vi "Producer main.vi"() -> ()   [LabVIEW 2017]
uses:
  Queue define.ctl
  <vilib>/FPGAPlugInAG/cRIO-9065/niLvFpga_Open_cRIO-9065.vi
  <vilib>/rvi/interface/common/dynamic/niFpgaDynamicAddResources.vi
  <vilib>/Utility/error.llb/Error Cluster From Error Code.vi
  <vilib>/rvi/errors/niLvFpgaAdjustHostInterfaceError.vi
  <vilib>/FPGAPlugInAG/Dynamic/niLvFpga_Run_Dynamic.vi
  <vilib>/FPGAPlugInAG/Dynamic/niLvFpga_Abort_Dynamic.vi
  <vilib>/rvi/interface/nirviOpenFPGA/nirviOpenFPGA.xnode
  FPGA Bitfiles/fpgaproject_FPGATarget_fpgamain2_8UW6JkLDP9I.lvbitx
  Fpga.vi
  <vilib>/rvi/interface/nirviMethod/nirviMethod.xnode
  <vilib>/rvi/interface/nirviReadWriteControl/nirviReadWriteControl.xnode
  NiFpgaLv.dll
  <vilib>/rvi/interface/Simulation/niFpgaSimulationCallBeginRW.vi
  <vilib>/FPGAPlugInAG/Dynamic/niLvFpga_StartFifo_Dynamic.vi
  <vilib>/rvi/errors/niLvFpgaMergeErrorWithErrorCode.vi
panel:
  in  "Die Casting?":bool
  out "Voltage Position":cluster{"Speed":dbl[], "Position":dbl[]}(graph)
  out "NO OFFSET Graph":cluster{"Speed":dbl[], "Position":dbl[]}(graph)
  out "OFFSET Graph":cluster{"Speed":dbl[], "Position":dbl[]}(graph)
  in  "程式終止":bool
  in  "Tab Control":enum32{"Speed / Position Setting"}(tab)
  in  "Speed/Position Set":bool
  in  "Y Speed":T1={"Speed 1"=1000.0, "Speed 2"=2000.0, "Speed 3"=3000.0, "Speed 4"=30000.0, "Speed 5"=50000.0, "Speed 6"=3000.0} {"Speed 6" step=100.0; "Speed 5" step=100.0; "Speed 4" step=100.0; "Speed 3" step=100.0; "Speed 2" step=100.0; "Speed 1" step=100.0}
  in  "X Position":T2={"Position 1"=100.0, "Position 2"=500.0, "Position 3"=1000.0, "Position 4"=1500.0, "Position 5"=2000.0, "Position 6"=2100.0} {"Position 6" step=100.0; "Position 5" step=100.0; "Position 4" step=100.0; "Position 3" step=100.0; "Position 2" step=100.0; "Position 1" step=100.0}
  in  "OFFSET":dbl=0.6 format="%#_13g"
  in  "Set Period":i64
  # "0.01mm"
  # "0.01mm"
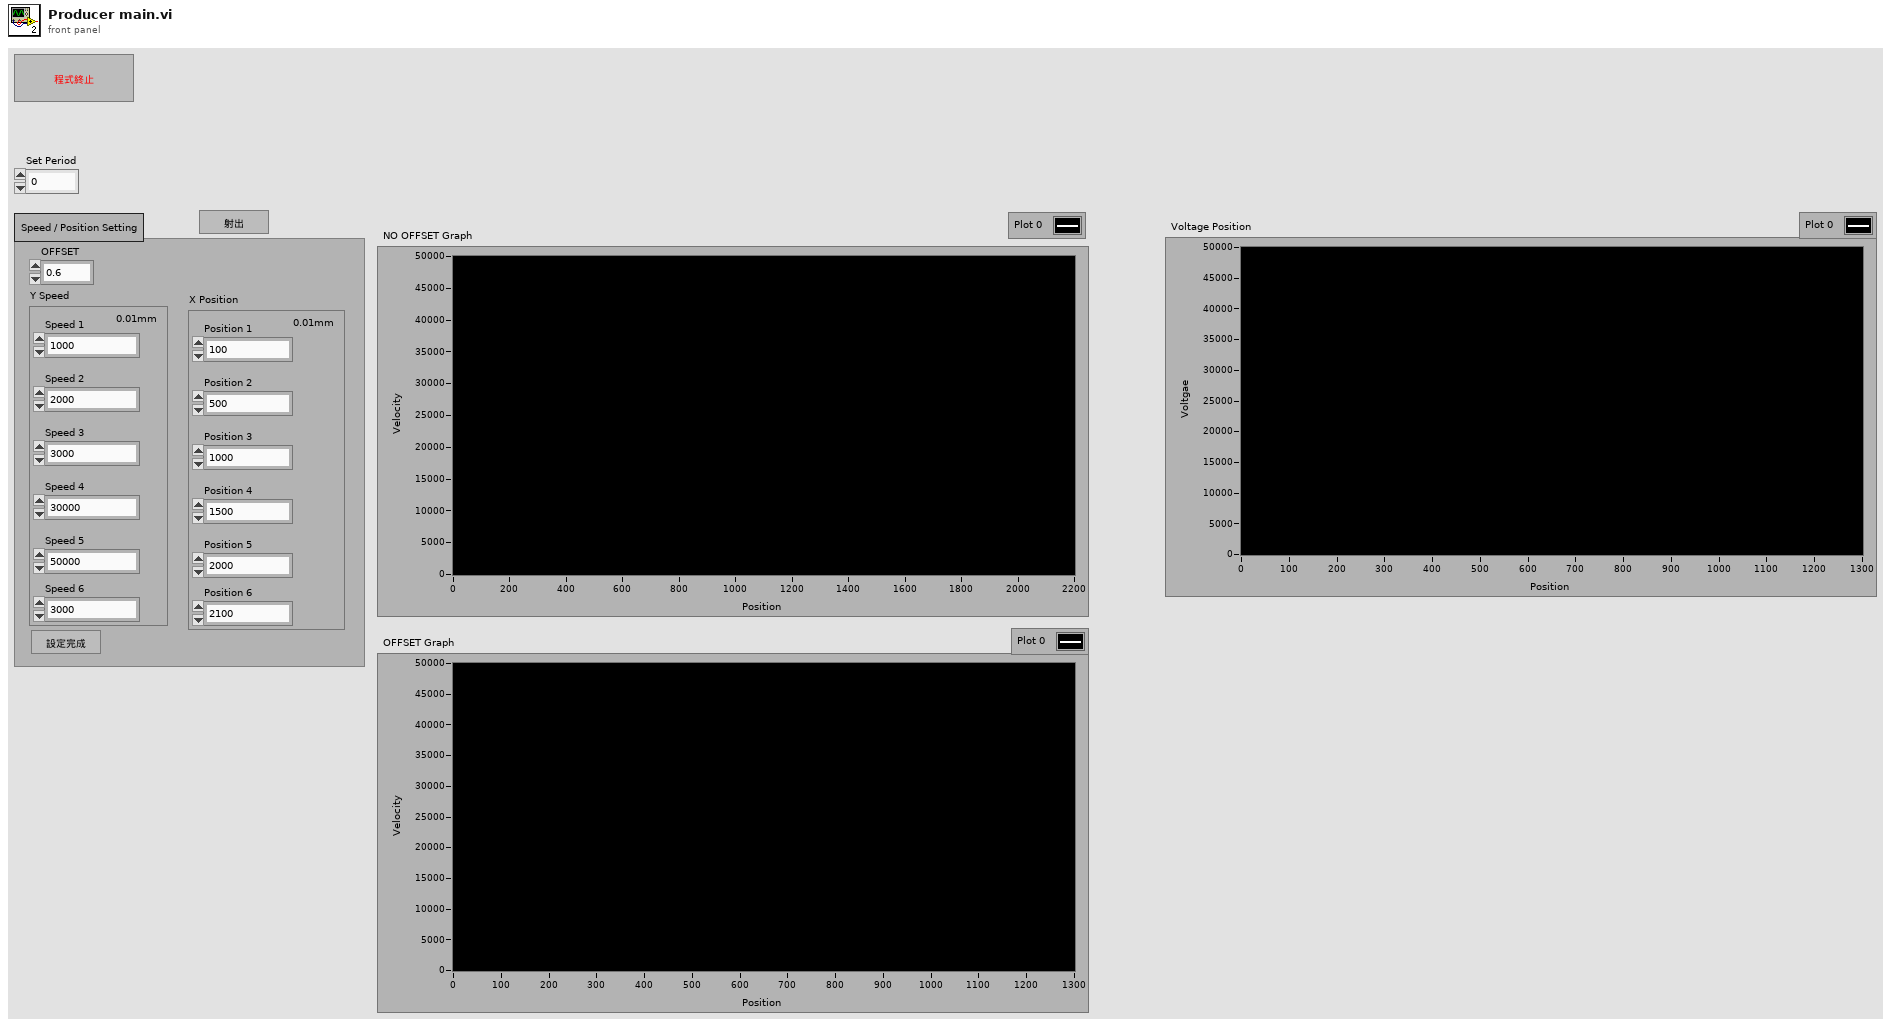
[diagram p1: front panel]
types:
  T1 = cluster{"Speed 1":dbl, "Speed 2":dbl, "Speed 3":dbl, "Speed 4":dbl, "Speed 5":dbl, "Speed 6":dbl}
  T2 = cluster{"Position 1":dbl, "Position 2":dbl, "Position 3":dbl, "Position 4":dbl, "Position 5":dbl, "Position 6":dbl}
  T3 = typedef "Queue define.ctl" = enum16{"Intiailze", "Curve Setting", "Die Casting", "stop"}
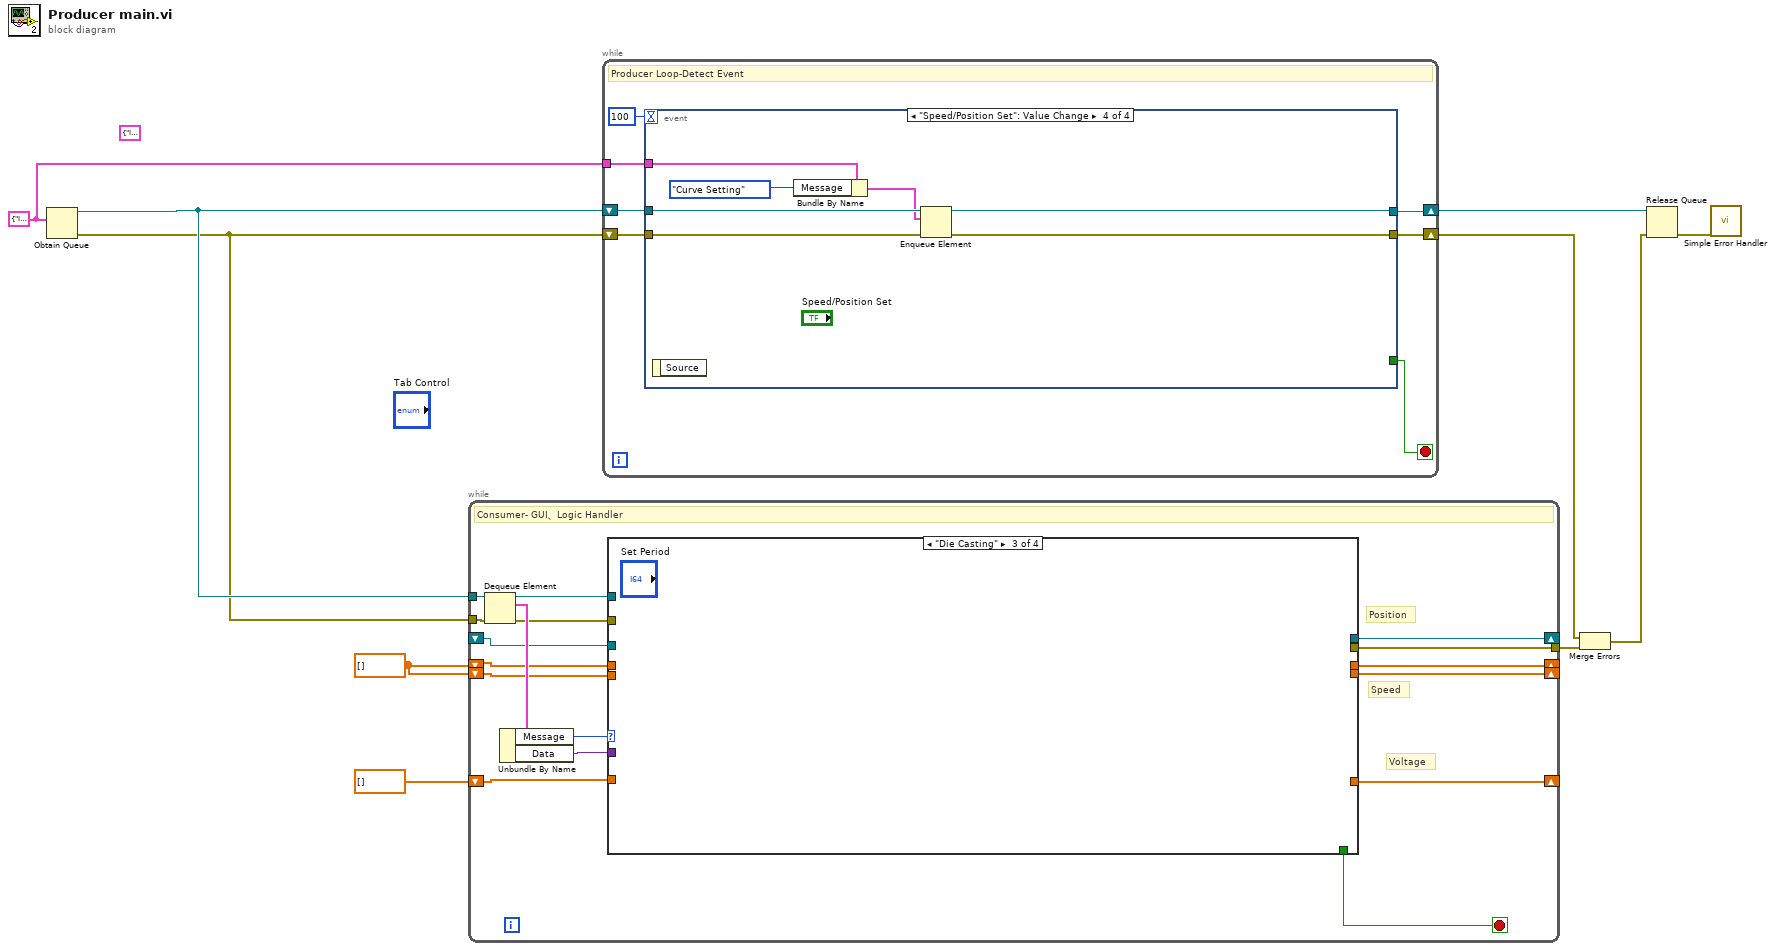
[diagram p0: block diagram]
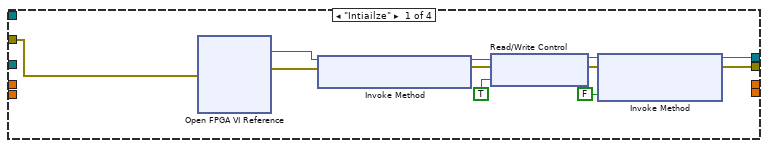
[diagram p2: hidden frame]
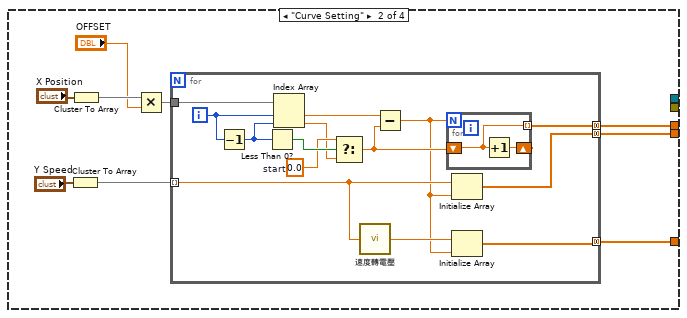
[diagram p3: hidden frame]
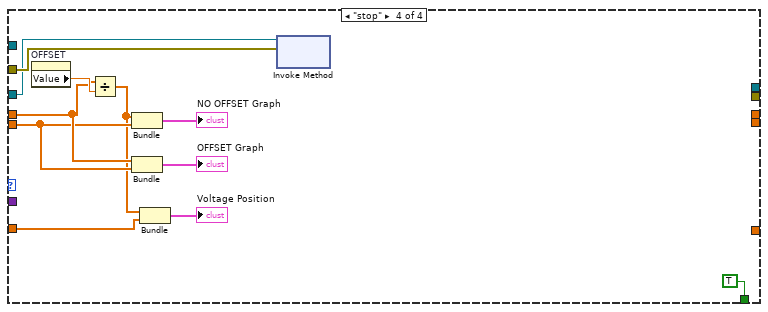
[diagram p4: hidden frame]
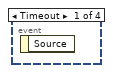
[diagram p5: hidden frame]
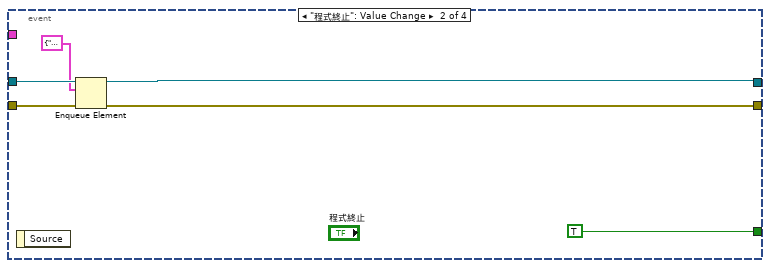
[diagram p6: hidden frame]
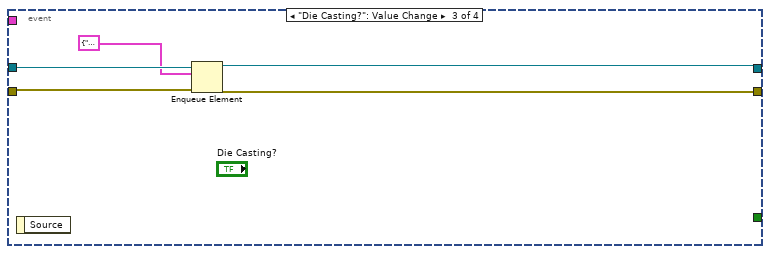
[diagram p7: hidden frame]
diagram:
  w6 = dbl[] []
  w1 = cluster{"Message":T3, "Data":variant} {"Message"=enum."Intiailze", "Data"=variant}
  (unwired) cluster{"Message":T3, "Data":variant} {"Message"=enum."Intiailze", "Data"=variant}
  n1 = Obtain Queue(element data type=w1) -> (queue out=w3:refnum<queue>, error out=w2:errorcluster)  [unwired: 4 in, 1 out]
  n2 = while {
    tunnel: w3 -> [w27]
    tunnel: w2 -> [w26]
    shift-right: [w21] -> _
    shift-left: _ -> [w19]
    shift-right: [w18] -> _
    shift-left: dbl[] [] -> [w15]
    shift-right: [w16] -> _
    shift-left: w6 -> [w14]
    shift-right: [w17] -> _
    shift-left: w6 -> [w13]
    tunnel: [w12] -> w10
    stop <- w11 stop-if-true
    # "Voltage"
    # "Speed"
    # "Position"
    # "Consumer- GUI、Logic Handler"
    n3 = Dequeue Element(queue=w27, error in (no error)=w26) -> (queue out=w23:refnum<queue>, element=w25:cluster{"Message":T3, "Data":variant}, error out=w22:errorcluster)  [unwired: 1 in, 1 out]
    n4 = Unbundle By Name(w25) -> ("Message"=w24:T3, "Data"=w20:variant)
    n5 = case shown="\"Die Casting\"" w24 {
      tunnel: w23 -> [_ _ _ _]
      tunnel: w22 -> [w28 _ _ w65]
      tunnel: [w32 _ _ _] -> w21
      tunnel: [w31 _ _ _] -> w12
      tunnel: w20 -> [_ _ _ _]
      tunnel: [_ w41 _ _] -> w16
      tunnel: [_ w40 _ _] -> w17
      tunnel: [_ w39 _ _] -> w18
      tunnel: w19 -> [_ _ _ w64]
      tunnel: w15 -> [_ _ _ w68]
      tunnel: w14 -> [_ _ _ w72]
      tunnel: w13 -> [_ _ _ w71]
      tunnel: [_ _ _ TRUE] -> w11
      frame "Intiailze" {
        n6 = xnode "Open FPGA VI Reference"("error in"=w28) -> ("FPGA VI Reference Out"=w29:refnum<k20>, "error out"=w30:errorcluster)  [unwired: 1 in]
        n7 = xnode "Invoke Method"("FPGA VI Reference In"=w29, "error in"=w30) -> ("FPGA VI Reference Out"=w36:refnum<k20>, "error out"=w35:errorcluster)
        n8 = xnode "Read/Write Control"("FPGA VI Reference In"=w36, "error in"=w35, "Position Reset"=TRUE) -> ("FPGA VI Reference Out"=w38:refnum<k20>, "error out"=w37:errorcluster)
        n9 = xnode "Invoke Method"("FPGA VI Reference In"=w38, "error in"=w37, "Wait Until Done (F)"=FALSE) -> ("FPGA VI Reference Out"=w32:refnum<k20>, "error out"=w31:errorcluster)
      }
      frame "Curve Setting" {
        n10 = Cluster To Array(cluster="Y Speed") -> (array=w43:dbl[])
        n11 = Cluster To Array(cluster="X Position") -> (array=w44:dbl[])
        n12 = Multiply(x=w44, y="OFFSET") -> (x*y=w45:dbl[])
        n13 = for {
          tunnel: w45 -> [w61]
          tunnel: w43 -> [w51] mode=indexing
          tunnel: [w54] -> w41 mode=concatenating
          tunnel: [w55] -> w40 mode=concatenating
          tunnel: [w48] -> w39 mode=concatenating
          i -> [w60]
          w57 = 0.0  # start
          n14 = Decrement(x=w60) -> (x-1=w59:i32)
          n15 = Less Than 0?(x=w59) -> (x < 0?=w58:bool)
          n16 = Index Array(array=w61, index #1=w60, index #2=w59) -> (element #1=w52:dbl, element #2=w56:dbl)
          n17 = Select(t=w57, s=w58, f=w56) -> (s? t:f=w53:dbl)
          n18 = call "速度轉電壓.vi"("Speed (0.1mm/s)"=w51) -> ("Voltage\nOutput"=w50:dbl)
          n19 = Subtract(x=w52, y=w53) -> (x-y=w49:dbl)
          n20 = for {
            N: w49 -> [_]
            shift-right: [w63] -> _
            shift-left: w53 -> [w62]
            tunnel: [w62] -> w54 mode=indexing
            n21 = Increment(x=w62) -> (x+1=w63:dbl)
          }
          n22 = Initialize Array(w51, w49) -> (w55:dbl[])
          n23 = Initialize Array(w50, w49) -> (w48:dbl[])
        }
      }
      frame "Die Casting" {
      }
      frame "stop" {
        n24 = property on="OFFSET" class="DigNum (strict)"() -> ("Value"=w74:dbl)  [unwired: 2 in, 2 out]
        n25 = Divide(x=w72, y=w74) -> (x/y=w69:dbl[])
        n26 = Bundle(w69, w71) -> (→"NO OFFSET Graph":cluster{dbl[], dbl[]})  [unwired: 1 in]
        n27 = Bundle(w72, w71) -> (→"OFFSET Graph":cluster{dbl[], dbl[]})  [unwired: 1 in]
        n28 = Bundle(w69, w68) -> (→"Voltage Position":cluster{dbl[], dbl[]})  [unwired: 1 in]
        n29 = xnode "Invoke Method"("FPGA VI Reference In"=w64, "error in"=w65) -> ()  [unwired: 2 out]
      }
    }
  }
  n30 = while {
    shift-right: [w77] -> w4
    shift-left: w3 -> [w80]
    shift-right: [w79] -> w8
    shift-left: w2 -> [w78]
    tunnel: w1 -> [w75]
    stop <- w81 stop-if-true
    # "Producer Loop-Detect Event"
    n31 = event shown="[3] \"Speed/Position Set\": Value Change" {
      selector: _ -> [_ _ _ _]
      dyn-events: _ -> [_ _ _ _]
      timeout: 100 -> [_ _ _ _]
      tunnel: [_ TRUE _ _] -> w81
      tunnel: w80 -> [_ w86 w92 w99]
      tunnel: w78 -> [_ w85 w91 w98]
      tunnel: [_ w83 w89 w97] -> w77
      tunnel: [_ w82 w88 w96] -> w79
      tunnel: w75 -> [_ _ _ w95]
      event Timeout {
        n32 = event-data() -> ()  [unwired: 1 in, 1 out]
      }
      event "程式終止": Value Change {
        n33 = event-data() -> ()  [unwired: 1 in, 1 out]
        n34 = Enqueue Element(queue=w86, element=cluster{"Message":T3, "Data":variant} {"Message"=enum."stop", "Data"=variant}, error in (no error)=w85) -> (queue out=w83:refnum<queue>, error out=w82:errorcluster)  [unwired: 1 in, 1 out]
      }
      event "Die Casting?": Value Change {
        n35 = event-data() -> ()  [unwired: 1 in, 1 out]
        n36 = Enqueue Element(queue=w92, element=cluster{"Message":T3, "Data":variant} {"Message"=enum."Die Casting", "Data"=variant}, error in (no error)=w91) -> (queue out=w89:refnum<queue>, error out=w88:errorcluster)  [unwired: 1 in, 1 out]
      }
      event "Speed/Position Set": Value Change {
        n37 = event-data() -> ()  [unwired: 1 in, 1 out]
        n38 = Bundle By Name(cluster=w95, "Message"=Queue_define."Curve Setting") -> (w93:cluster{"Message":T3, "Data":variant})
        n39 = Enqueue Element(queue=w99, element=w93, error in (no error)=w98) -> (queue out=w97:refnum<queue>, error out=w96:errorcluster)  [unwired: 1 in, 1 out]
      }
    }
  }
  n40 = Merge Errors(w8, w10) -> (w9:errorcluster)
  n41 = Release Queue(queue=w4, error in (no error)=w9) -> (error out=w7:errorcluster)  [unwired: 1 in, 2 out]
  n42 = call <vilib>:"Simple Error Handler.vi"("error in (no error)"=w7) -> ()  [unwired: 4 in, 5 out]
